vi "Laser Damage Scan Alpha.vi"(7 "Calling VI Ref":refnum<vi>) -> ()   [LabVIEW 2020]
uses:
  <vilib>/vision/Image Controls.llb/IMAQ Image.ctl
  <vilib>/Utility/miscctls.llb/LVPointTypeDef.ctl
  Display Module/Display Module Custom Controls/ROI Descriptor.ctl
  <vilib>/DAQmx/write.llb/DAQmx Write (Analog 1D Wfm NChan NSamp).vi
  <vilib>/Instr/_visa.llb/VISA Configure Serial Port (Instr).vi
  <vilib>/DAQmx/create/channels.llb/DAQmx Create Channel (AO-Voltage-Basic).vi
  <vilib>/DAQmx/configure/timing.llb/DAQmx Timing (Sample Clock).vi
  <vilib>/DAQmx/miscellaneous.llb/DAQmx Fill In Error Info.vi
  <resource>/objmgr/daqmx.rc
  <vilib>/measure/NI_MABase.lvlib
panel:
  in  "Active Image":u16(ring) items=["IDS-Camera-Primary-2", "IDS-Camera-Primary-3", "IDS-Camera-Primary-4"]
  in  "Manual Shutter":bool
  out "Current Exposure Time (s)":dbl=1.0 max=100.0 format="%.1f"
  out "Scan Error":bool
  in  "Scan Rate (Hz)":dbl=1.0 max=100.0
  in  "Exposure Time (s)":i32=1 max=100
  out "Shutter Error":bool
  in  "Ablate":bool
  out "Waveform Graph":waveform(dbl)[](graph)=[{"t0"=timestamp(0 s since 1904-01-01), "dt"=0.001, "Y"=array[100000 elements]}, {"t0"=timestamp(0 s since 1904-01-01), "dt"=0.001, "Y"=array[100000 elements]}, {"t0"=timestamp(0 s since 1904-01-01), "dt"=0.001, "Y"=array[100000 elements]}]
  in  "Quit":bool
  out "ROI Error":bool
  out "ROI Data":i32[](array[numeric])
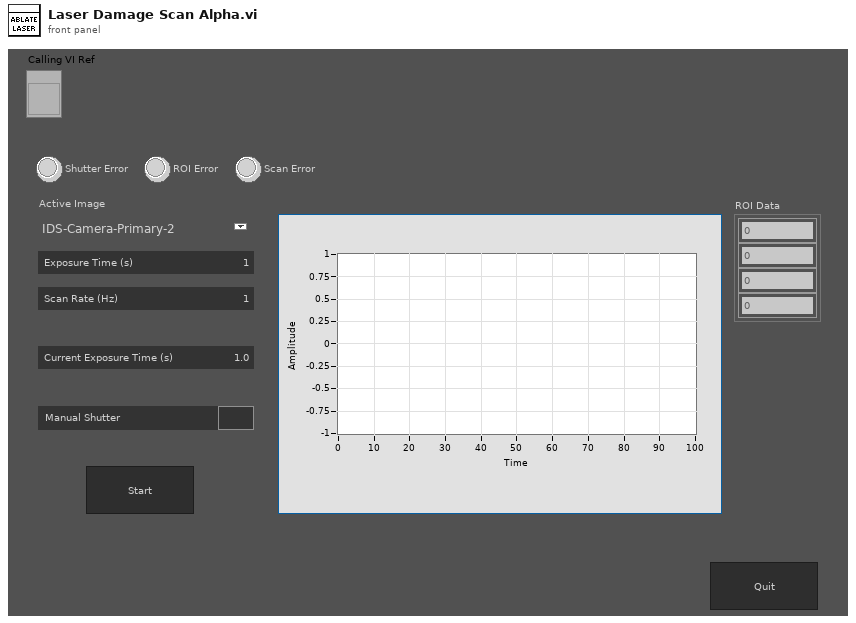
[diagram p1: front panel]
types:
  T1 = enum16{"Always On", "Always Off", "Off While Running"}
  T2 = typedef "LVPointTypeDef.ctl" = cluster{"Horizontal":i16, "Vertical":i16}
  T3 = cluster{"Vx":dbl, "Xfreq":dbl, "Xoff":dbl, "Yfreq":dbl, "Vy":dbl, "Yoff":dbl}
  T4 = typedef "IMAQ Image.ctl" = refnum<image>
  T5 = typedef "ROI Descriptor.ctl" = cluster{"Global Rectangle":i32[], "Contours":cluster{"Contour Type":u32, "ROI Type":u32, "Points":i32[]}[]}
  T6 = cluster{"Waveform Type":u16, "Amplitude":dbl, "Frequency":dbl, "Phase":dbl, "Offset":dbl}
  T7 = cluster{"Waveform Type":u16, "Amplitude":dbl, "Frequency":dbl, "Phase":dbl, "Offset":dbl}[]
  T8 = typedef "LVRectTypeDef.ctl" = cluster{"Left":i16, "Top":i16, "Right":i16, "Bottom":i16}
  T9 = typedef "LVBoundsTypeDef.ctl" = cluster{"Width":u32, "Height":u32}
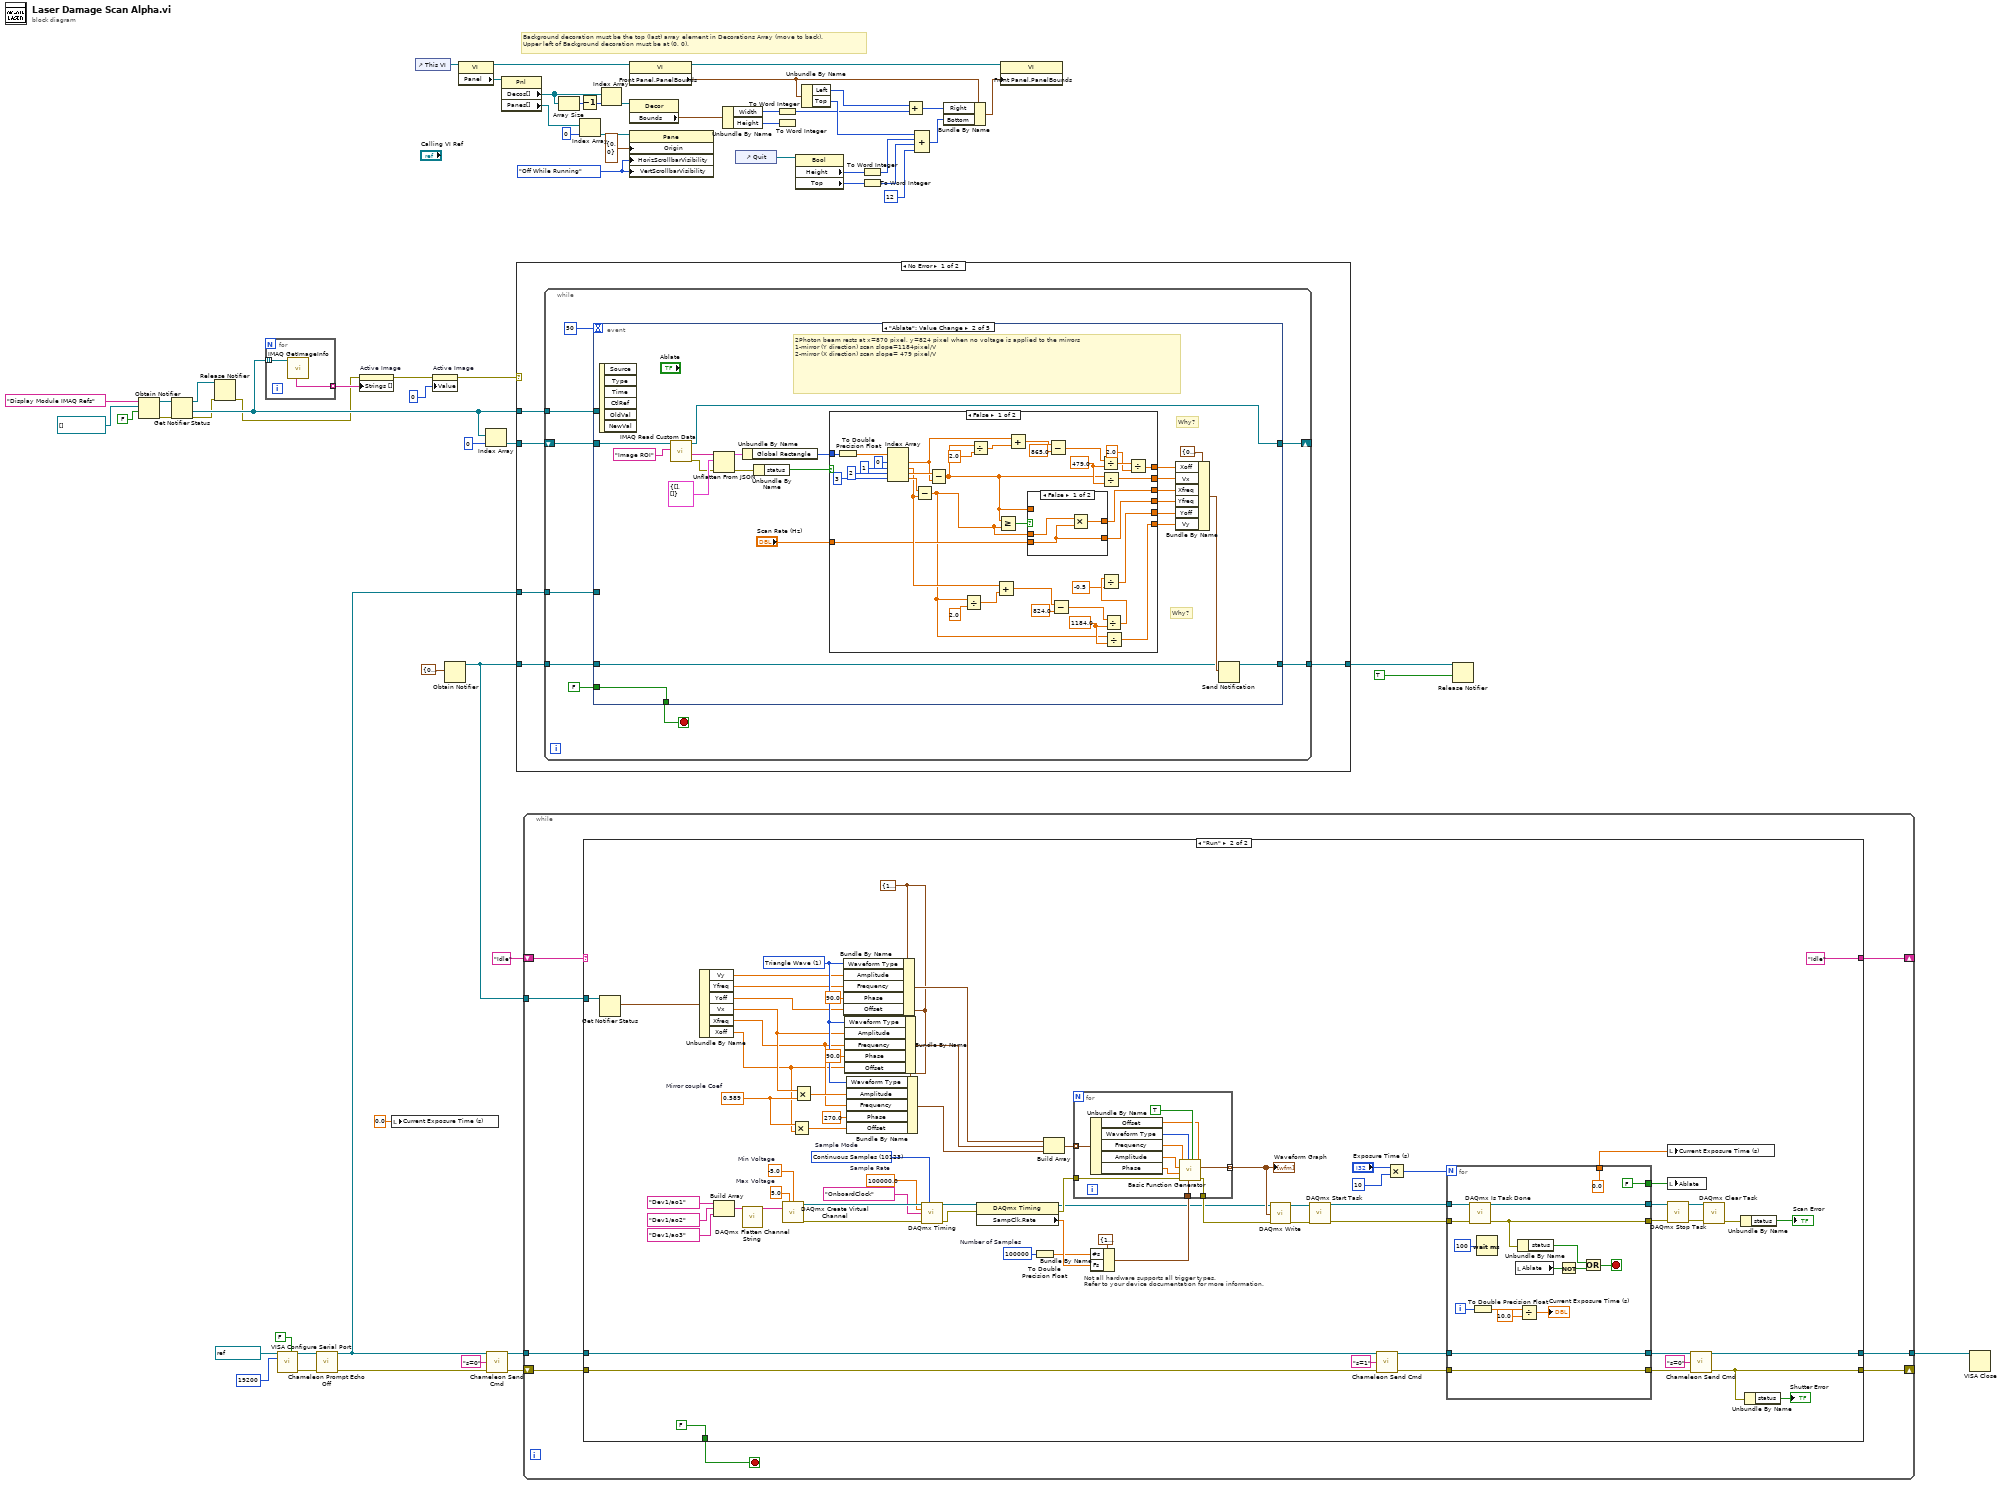
[diagram p0: block diagram]
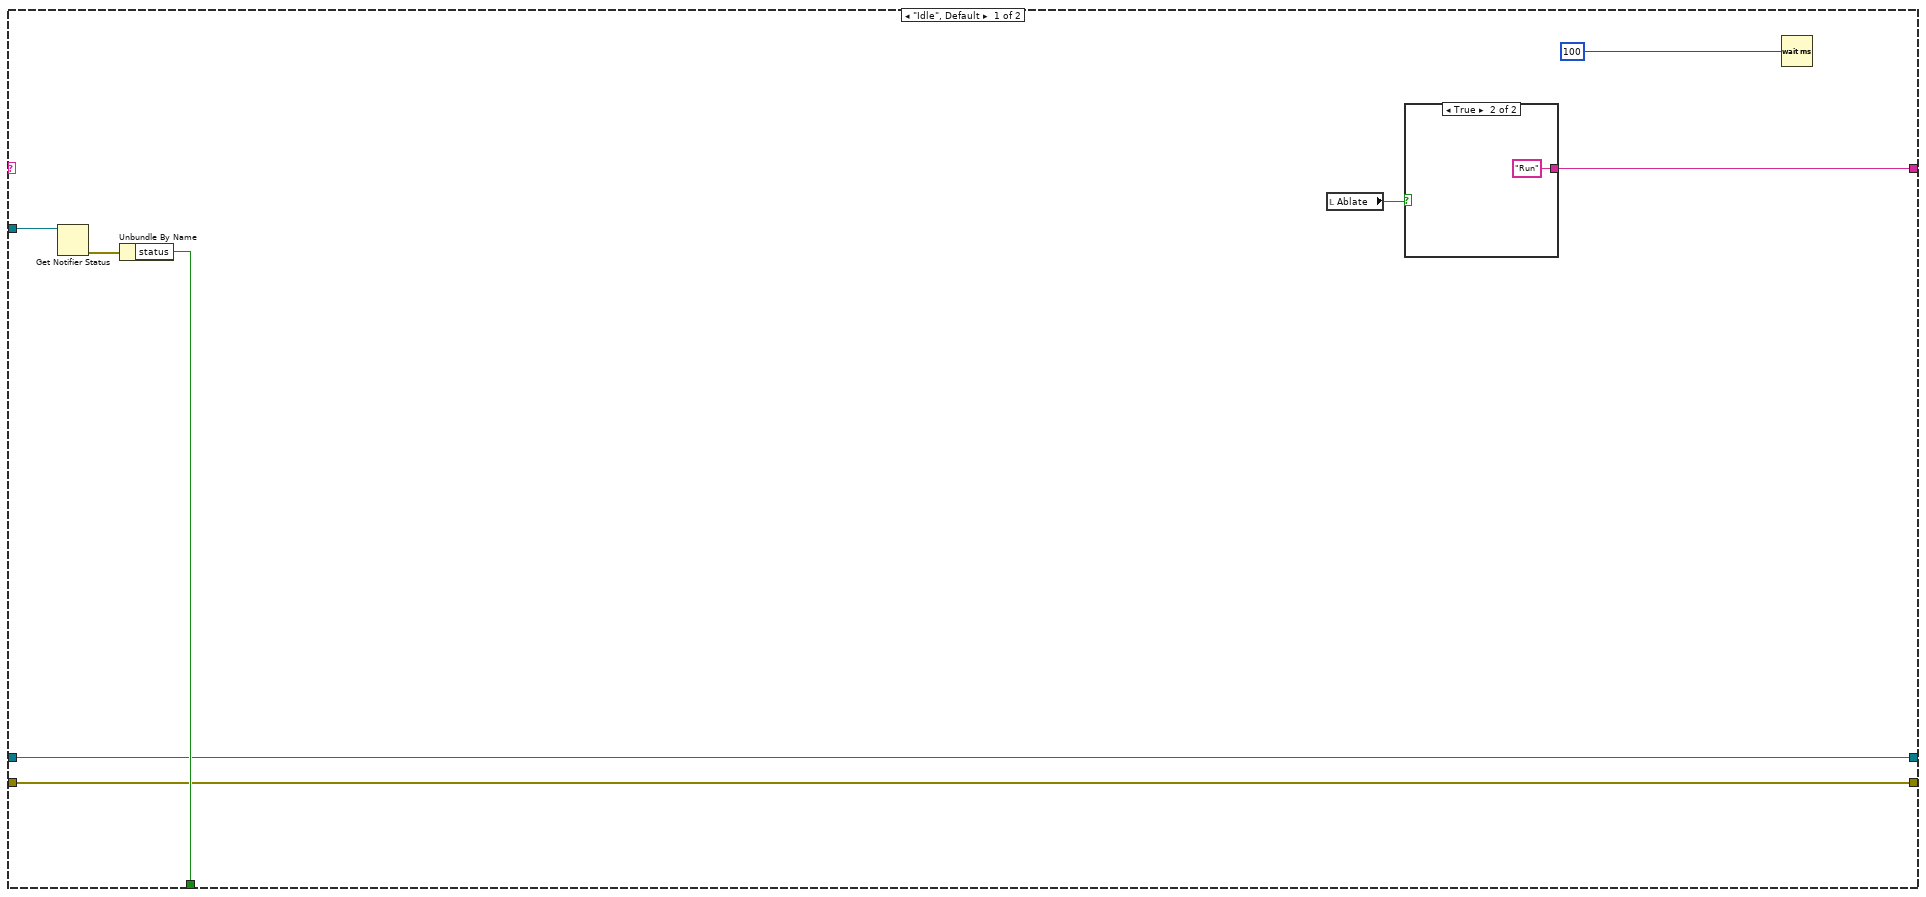
[diagram p2: hidden frame]
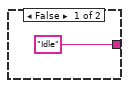
[diagram p3: hidden frame]
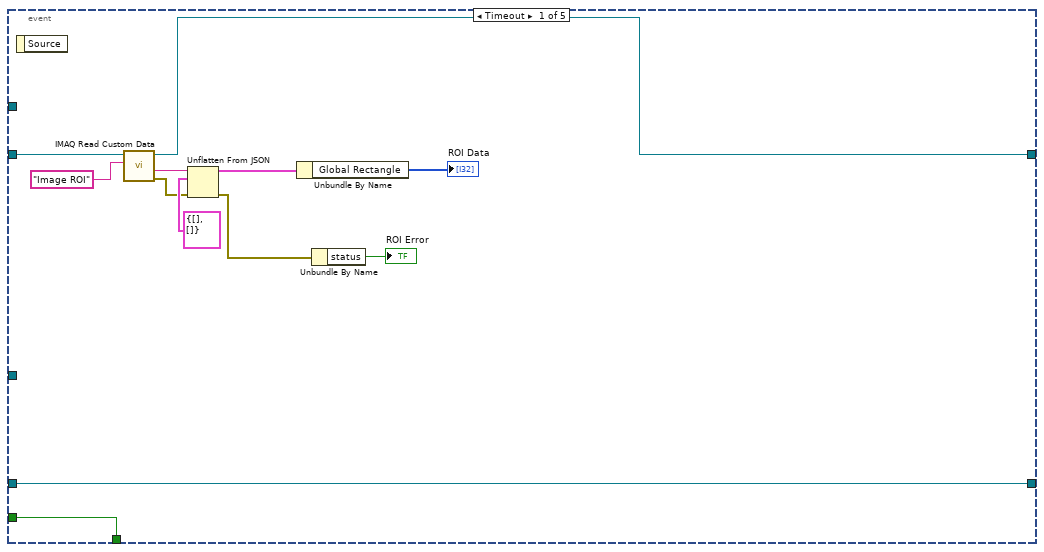
[diagram p4: hidden frame]
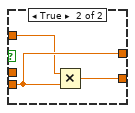
[diagram p5: hidden frame]
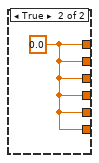
[diagram p6: hidden frame]
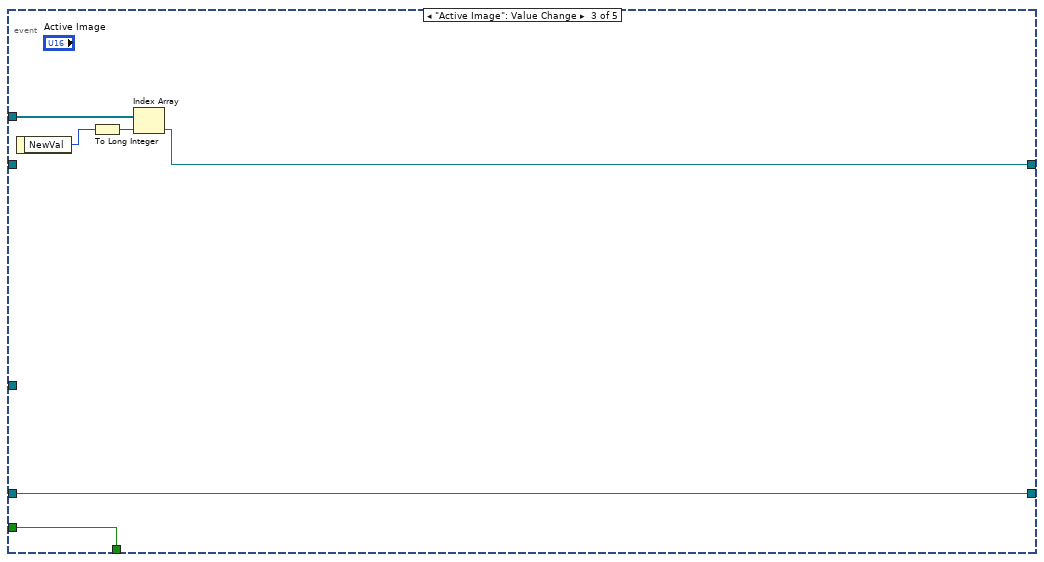
[diagram p7: hidden frame]
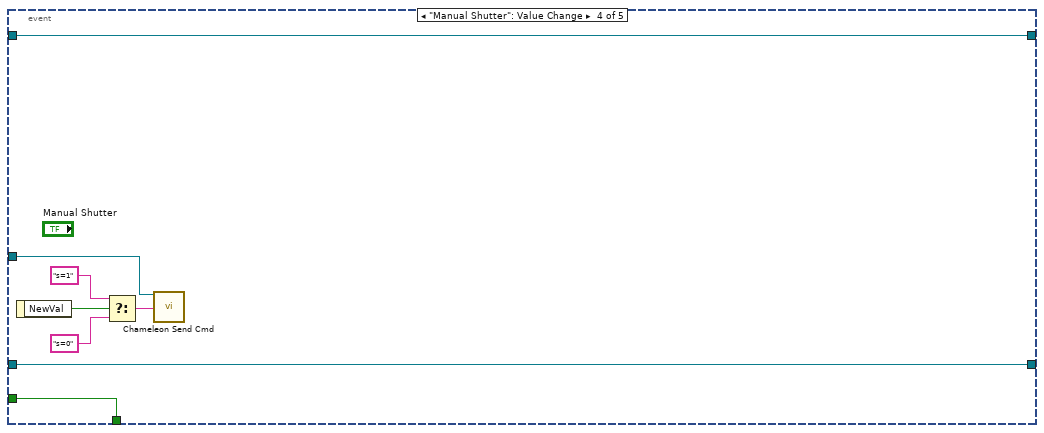
[diagram p8: hidden frame]
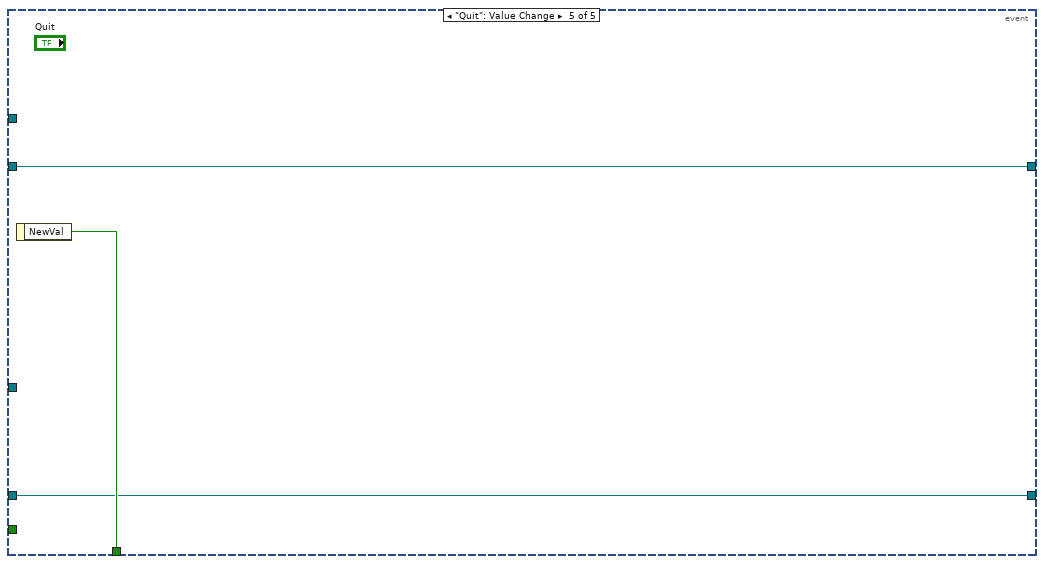
[diagram p9: hidden frame]
diagram:
  w13 = T1."Off While Running" ("Vertical Scrollbar Visibility")
  # "Background decoration must be the top (last) array element in Decorations Array (move to back).\nUpper left of Background decoration must be at (0, 0)."
  n1 = Obtain Notifier(name (unnamed)="Display Module IMAQ Refs", notification data type=T4[] [], create if not found? (T)=FALSE) -> (notifier out=w61:refnum<notifier>, error out=w60:errorcluster)  [unwired: 1 in, 1 out]
  n2 = Get Notifier Status(notifier=w61, error in (no error)=w60) -> (notifier out=w49:refnum<notifier>, current notification=w54:T4[], error out=w48:errorcluster)  [unwired: 2 out]
  n3 = Release Notifier(notifier=w49, error in (no error)=w48) -> (error out=w47:errorcluster)  [unwired: 1 in, 2 out]
  n4 = for {
    tunnel: w54 -> [w63] mode=indexing
    tunnel: [w62] -> w53 mode=indexing
    n5 = call "IMAQ GetImageInfo"("Image"=w63) -> ("Image Name"=w62:string)  [unwired: 3 in, 7 out]
  }
  n6 = call-poly "VISA Configure Serial Port"("VISA resource name"=refnum<visa-resource-name> "COM13" ("VISA Ref"), "Enable Termination\nChar (T)"=FALSE ("Enable Termination\nChar (T)"), "baud rate (9600)"=u32 19200) -> ("VISA resource name out"=w38:refnum<visa-resource-name>, "error out"=w37:errorcluster)  [unwired: 11 in]
  n7 = call "Chameleon Prompt Echo Off.vi"("VISA Ref"=w38, "Error In"=w37) -> ("VISA Ref Out"=w31:refnum<visa-resource-name>, "Error Out"=w33:errorcluster)  [unwired: 12 in]
  n8 = property on="Active Image" class="Ring (strict)"(error in=w47, "Strings []"=w53) -> (error out=w51:errorcluster)  [unwired: 1 in, 1 out]
  n9 = local write "Current Exposure Time (s)"(0.0 ("Current Exposure Time (s)")) -> ()
  n10 = control-ref of="This VI"() -> (w5:refnum<vi>)
  n11 = property on="Active Image" class="Ring (strict)"(error in=w51, "Value"=u16 0) -> (error out=w50:errorcluster)  [unwired: 1 in, 1 out]
  n12 = Obtain Notifier(notification data type=T3 {"Vx"=0.25, "Xfreq"=1.0, "Xoff"=0.1, "Yfreq"=1.0, "Vy"=0.25, "Yoff"=0.1} ("Cluster")) -> (notifier out=w43:refnum<notifier>)  [unwired: 3 in, 2 out]
  n13 = property class="VI"(reference=w5) -> (reference out=w14:refnum<vi>, "Panel"=w6:refnum<vi>)  [unwired: 1 in, 1 out]
  n14 = Index Array(array=w54, index=0) -> (element=w55:T4)
  n15 = call "Chameleon Send Cmd.vi"("VISA Ref"=w31, "Command"="s=0", "Error In"=w33) -> ("VISA Ref Out"=w34:refnum<visa-resource-name>, "Error Out"=w32:errorcluster)  [unwired: 10 in, 1 out]
  n16 = property class="Pnl"(reference=w6) -> ("Decos[]"=w4:refnum<vi>[], "Panes[]"=w10:refnum<vi>[])  [unwired: 1 in, 2 out]
  n17 = case shown="No Error" w50 {
    tunnel: w55 -> [w68 _]
    tunnel: w54 -> [w67 _]
    tunnel: w43 -> [w66 w172]
    tunnel: [w65 w172] -> w45
    tunnel: w31 -> [w64 _]
    frame No Error {
      n18 = while {
        shift-right: [w74] -> _
        shift-left: w68 -> [w75]
        tunnel: w67 -> [w76]
        tunnel: w66 -> [w71]
        tunnel: [w70] -> w65
        tunnel: w64 -> [w69]
        stop <- w72 stop-if-true
        n19 = event shown="[1] \"Ablate\": Value Change" {
          selector: _ -> [_ _ _ _ _]
          dyn-events: _ -> [_ _ _ _ _]
          timeout: 50 -> [_ _ _ _ _]
          tunnel: w76 -> [_ _ w159 _ _]
          tunnel: w75 -> [w84 w106 _ w166 w170]
          tunnel: [w83 w105 w156 w166 w170] -> w74
          tunnel: FALSE -> [w80 w104 w160 w168 _]
          tunnel: [w80 w104 w160 w168 w171] -> w72
          tunnel: w71 -> [w79 w97 w155 w167 w169]
          tunnel: [w79 w96 w155 w167 w169] -> w70
          tunnel: w69 -> [_ _ _ w161 _]
          event Timeout {
            n20 = event-data() -> ()  [unwired: 1 in, 1 out]
            n21 = call "IMAQ Read Custom Data"("Key"="Image ROI", "Image"=w84) -> ("error out"=w85:errorcluster, "Custom Data Out"=w88:string, "Image (duplicate)"=w83:T4)  [unwired: 7 in]
            n22 = Unflatten From JSON(JSON string=w88, type and defaults=T5 {"Global Rectangle"=[], "Contours"=[]} ("Image ROI Descriptor"), error in (no error)=w85) -> (value=w86:T5, error out=w82:errorcluster)  [unwired: 4 in]
            n23 = Unbundle By Name(w86) -> ("Global Rectangle"=→"ROI Data":i32[])
            n24 = Unbundle By Name(w82) -> ("status"=→"ROI Error":bool)
          }
          event "Ablate": Value Change {
            # "Why?"
            # "Why?"
            # "2Photon beam rests at x=870 pixel, y=824 pixel when no voltage is applied to the mirrors\n1-mirror (Y direction) scan slope=1184pixel/V\n2-mirror (X direction) scan slope= 479 pixel/V"
            n25 = event-data() -> ()  [unwired: 1 in, 6 out]
            n26 = call "IMAQ Read Custom Data"("Key"="Image ROI", "Image"=w106) -> ("error out"=w107:errorcluster, "Custom Data Out"=w110:string, "Image (duplicate)"=w105:T4)  [unwired: 7 in]
            n27 = Unflatten From JSON(JSON string=w110, type and defaults=T5 {"Global Rectangle"=[], "Contours"=[]} ("Image ROI Descriptor"), error in (no error)=w107) -> (value=w108:T5, error out=w92:errorcluster)  [unwired: 4 in]
            n28 = Unbundle By Name(w108) -> ("Global Rectangle"=w93:i32[])
            n29 = Unbundle By Name(w92) -> ("status"=w91:bool)
            n30 = case shown="False" w91 {
              tunnel: w93 -> [w147 _]
              tunnel: [w136 w154] -> w102
              tunnel: [w131 w154] -> w101
              tunnel: "Scan Rate (Hz)" -> [w129 _]
              tunnel: [w128 w154] -> w100
              tunnel: [w127 w154] -> w99
              tunnel: [w125 w154] -> w95
              tunnel: [w121 w154] -> w94
              frame False {
                w133 = 1184.0 ("y")
                w134 = 479.0 ("y")
                n31 = To Double Precision Float(number=w147) -> (double precision float=w120:dbl[])
                n32 = Index Array(array=w120, index #1=0 ("index"), index #2=1 ("index"), index #3=2 ("index"), index #4=3 ("index")) -> (element #1=w138:dbl, element #2=w137:dbl, element #3=w142:dbl, element #4=w140:dbl)
                n33 = Subtract(x=w140, y=w137) -> (x-y=w112:dbl)
                n34 = Subtract(x=w142, y=w138) -> (x-y=w116:dbl)
                n35 = Divide(x=w112, y=2.0) -> (x/y=w115:dbl)
                n36 = Divide(x=w116, y=2.0) -> (x/y=w119:dbl)
                n37 = Add(x=w137, y=w115) -> (x+y=w114:dbl)
                n38 = Greater Or Equal?(x=w116, y=w112) -> (x >= y?=w130:bool)
                n39 = Add(x=w138, y=w119) -> (x+y=w118:dbl)
                n40 = case shown="False" w130 {
                  tunnel: w129 -> [w150 w152]
                  tunnel: [w150 w153] -> w128
                  tunnel: w112 -> [w148 _]
                  tunnel: [w149 w152] -> w127
                  tunnel: w116 -> [_ w151]
                  frame False {
                    n41 = Multiply(x=w148, y=w150) -> (x*y=w149:dbl)
                  }
                  frame True {
                    n42 = Multiply(x=w151, y=w152) -> (x*y=w153:dbl)
                  }
                }
                n43 = Subtract(x=w118, y=865.0) -> (x-y=w117:dbl)
                n44 = Subtract(x=w114, y=824.0) -> (x-y=w113:dbl)
                n45 = Divide(x=w117, y=w134) -> (x/y=w126:dbl)
                n46 = Divide(x=w116, y=w134) -> (x/y=w136:dbl)
                n47 = Divide(x=w113, y=w133) -> (x/y=w123:dbl)
                n48 = Divide(x=w123, y=-0.5) -> (x/y=w121:dbl)
                n49 = Divide(x=w112, y=w133) -> (x/y=w131:dbl)
                n50 = Divide(x=w126, y=2.0) -> (x/y=w125:dbl)
              }
              frame True {
                w154 = 0.0
              }
            }
            n51 = Bundle By Name(cluster=T3 {"Vx"=0.25, "Xfreq"=1.0, "Xoff"=0.1, "Yfreq"=1.0, "Vy"=0.25, "Yoff"=0.1} ("Cluster"), "Xoff"=w95, "Vx"=w102, "Xfreq"=w99, "Yfreq"=w100, "Yoff"=w94, "Vy"=w101) -> (w98:T3)
            n52 = Send Notification(notification=w98, notifier=w97) -> (notifier out=w96:refnum<notifier>)  [unwired: 1 in, 1 out]
          }
          event "Active Image": Value Change {
            n53 = event-data() -> ("NewVal"=w158:u16)  [unwired: 1 in]
            n54 = To Long Integer(number=w158) -> (32bit integer=w157:i32)
            n55 = Index Array(array=w159, index=w157) -> (element=w156:T4)
          }
          event "Manual Shutter": Value Change {
            n56 = event-data() -> ("NewVal"=w165:bool)  [unwired: 1 in]
            n57 = Select(t="s=1" ("Command"), s=w165, f="s=0" ("Command")) -> (s? t:f=w162:string)
            n58 = call "Chameleon Send Cmd.vi"("VISA Ref"=w161, "Command"=w162) -> ()  [unwired: 11 in, 3 out]
          }
          event "Quit": Value Change {
            n59 = event-data() -> ("NewVal"=w171:bool)  [unwired: 1 in]
          }
        }
      }
    }
    frame Error {
    }
  }
  n60 = while {
    tunnel: w43 -> [w179]
    shift-right: [w178] -> _
    shift-left: "Idle" -> [w177]
    shift-right: [w173] -> _
    shift-left: w32 -> [w176]
    tunnel: w34 -> [w175]
    tunnel: [w174] -> w36
    stop <- w180 stop-if-true
    n61 = case shown="\"Run\"" w177 {
      tunnel: [w186 FALSE] -> w180
      tunnel: w179 -> [w188 w216]
      tunnel: [w184 "Idle"] -> w178
      tunnel: w176 -> [w181 w207]
      tunnel: w175 -> [w182 w208]
      tunnel: [w182 w206] -> w174
      tunnel: [w181 w205] -> w173
      frame "Idle", Default {
        n62 = Get Notifier Status(notifier=w188) -> (error out=w187:errorcluster)  [unwired: 1 in, 4 out]
        n63 = Unbundle By Name(w187) -> ("status"=w186:bool)
        n64 = local read "Ablate"() -> (w185:bool)
        n65 = case shown="True" w185 {
          tunnel: ["Idle" "Run"] -> w184
          frame False {
          }
          frame True {
          }
        }
        n66 = Wait (ms)(milliseconds to wait=u32 100) -> ()  [unwired: 1 out]
      }
      frame "Run" {
        w242 = 100000  # Number of Samples
        w220 = 0.589  # Mirror couple Coef
        w251 = 5.0  # Max Voltage
        w252 = -5.0  # Min Voltage
        w225 = u16 1 items=["Sine Wave", "Triangle Wave", "Square Wave", "Sawtooth Wave"] ("Waveform Type")
        w226 = T6 {"Waveform Type"=1, "Amplitude"=0.25, "Frequency"=1.0, "Phase"=180.0, "Offset"=0.1} ("Cluster")
        w253 = 100000.0  # Sample Rate
        w259 = 10123 items=["Finite Samples"=10178, "Continuous Samples"=10123, "Hardware Timed Single Point"=12522]  # Sample Mode
        # "Not all hardware supports all trigger types.\nRefer to your device documentation for more information."
        n67 = Get Notifier Status(notifier=w216) -> (current notification=w215:T3)  [unwired: 1 in, 4 out]
        n68 = Unbundle By Name(w215) -> ("Vy"=w214:dbl, "Yfreq"=w213:dbl, "Yoff"=w212:dbl, "Vx"=w211:dbl, "Xfreq"=w210:dbl, "Xoff"=w209:dbl)
        n69 = Build Array(tag "Dev1/ao1" ("Physical Channel(s)"), tag "Dev1/ao2" ("Physical Channel(s)"), tag "Dev1/ao3" ("Physical Channel(s)")) -> (w234:tag[])
        n70 = call <vilib>:"DAQmx Flatten Channel String.vi"("names in"=w234) -> ("names out"=w231:string)  [unwired: 13 in, 1 out]
        n71 = call-poly <vilib>:"DAQmx Create Virtual Channel.vi"("maximum value"=w251, "minimum value"=w252, "physical channels"=w231) -> ("task out"=w257:refnum<k21>, "error out"=w258:errorcluster)  [unwired: 11 in]
        n72 = Multiply(x=w220, y=w209) -> (x*y=w219:dbl)
        n73 = Multiply(x=w211, y=w220) -> (x*y=w221:dbl)
        n74 = Bundle By Name(cluster=w226, "Waveform Type"=w225, "Amplitude"=w214, "Frequency"=w213, "Phase"=90.0, "Offset"=w212) -> (w229:T6)
        n75 = Bundle By Name(cluster=w226, "Waveform Type"=w225, "Amplitude"=w211, "Frequency"=w210, "Phase"=90.0, "Offset"=w209) -> (w228:T6)
        n76 = Bundle By Name(cluster=w226, "Waveform Type"=w225, "Amplitude"=w221, "Frequency"=w210, "Phase"=270.0, "Offset"=w219) -> (w227:T6)
        n77 = call-poly <vilib>:"DAQmx Timing.vi"("task/channels in"=w257, "sample mode"=w259, "rate"=w253, "source"=tag "OnboardClock" ("Sample Clock Source"), "error in"=w258) -> ("task out"=w261:refnum<k21>, "error out"=w260:errorcluster)  [unwired: 9 in]
        n78 = property class="DAQmx Timing"(reference=w261, error in=w260) -> (reference out=w236:refnum<k21>, error out=w237:errorcluster, "SampClk.Rate"=w249:dbl)
        n79 = To Double Precision Float(number=w242) -> (double precision float=w243:dbl)
        n80 = Build Array(w229, w228, w227) -> (w230:T7)
        n81 = Bundle By Name(cluster=cluster{"Fs":dbl, "#s":dbl} {"Fs"=1000.0, "#s"=1000.0} ("sampling info"), "#s"=w243, "Fs"=w249) -> (w248:cluster{"Fs":dbl, "#s":dbl})
        n82 = for {
          tunnel: w237 -> [w289]
          tunnel: w248 -> [w288]
          tunnel: [w287] -> w245
          tunnel: w230 -> [w286] mode=indexing
          tunnel: [w282] -> w244 mode=indexing
          n83 = Unbundle By Name(w286) -> ("Offset"=w279:dbl, "Waveform Type"=w285:u16, "Frequency"=w284:dbl, "Amplitude"=w283:dbl, "Phase"=w281:dbl)
          n84 = call <vilib>:"Basic Function Generator.vi"("offset"=w279, "reset signal"=TRUE, "sampling info"=w288, "signal type"=w285, "error in (no error)"=w289, "phase"=w281, "amplitude"=w283, "frequency"=w284) -> ("error out"=w287:errorcluster, "signal out"=w282:waveform(dbl))  [unwired: 1 in, 1 out]
        }
        "Waveform Graph" <- w244
        n85 = call-poly <vilib>:"DAQmx Write.vi"("task/channels in"=w236, "data"=w244, "error in"=w245) -> ("task out"=w247:refnum<k21>, "error out"=w246:errorcluster)  [unwired: 10 in, 1 out]
        n86 = call <vilib>:"DAQmx Start Task.vi"("task/channels in"=w247, "error in"=w246) -> ("task out"=w256:refnum<k21>, "error out"=w255:errorcluster)  [unwired: 12 in]
        n87 = call "Chameleon Send Cmd.vi"("VISA Ref"=w208, "Command"="s=1", "Error In"=w207) -> ("VISA Ref Out"=w200:refnum<visa-resource-name>, "Error Out"=w199:errorcluster)  [unwired: 10 in, 1 out]
        n88 = Multiply(x="Exposure Time (s)", y=10) -> (x*y=w195:i32)
        n89 = for {
          N: w195 -> [_]
          tunnel: w256 -> [w278]
          tunnel: w255 -> [w277]
          tunnel: [w275] -> w238
          tunnel: [w276] -> w239
          tunnel: [w272] -> w201
          tunnel: w200 -> [w272]
          tunnel: w199 -> [w271]
          tunnel: [w271] -> w198
          tunnel: [FALSE] -> w194
          tunnel: [0.0] -> w191
          i -> [w266]
          stop <- w268 stop-if-true
          n90 = call <vilib>:"DAQmx Is Task Done.vi"("task/channels in"=w278, "error in"=w277) -> ("task out"=w276:refnum<k21>, "error out"=w275:errorcluster)  [unwired: 11 in, 1 out]
          n91 = To Double Precision Float(number=w266) -> (double precision float=w265:dbl)
          n92 = Wait (ms)(milliseconds to wait=u32 100) -> ()  [unwired: 1 out]
          n93 = local read "Ablate"() -> (w274:bool)
          n94 = Unbundle By Name(w275) -> ("status"=w270:bool)
          n95 = Divide(x=w265, y=10.0) -> (x/y=→"Current Exposure Time (s)":dbl)
          n96 = Not(x=w274) -> (.not. x?=w269:bool)
          n97 = Or(x=w270, y=w269) -> (x .or. y?=w268:bool)
        }
        n98 = local write "Current Exposure Time (s)"(w191) -> ()
        n99 = local write "Ablate"(w194) -> ()
        n100 = call <vilib>:"DAQmx Stop Task.vi"("task/channels in"=w239, "error in"=w238) -> ("task out"=w241:refnum<k21>, "error out"=w240:errorcluster)  [unwired: 12 in]
        n101 = call "Chameleon Send Cmd.vi"("VISA Ref"=w201, "Command"="s=0", "Error In"=w198) -> ("VISA Ref Out"=w206:refnum<visa-resource-name>, "Error Out"=w205:errorcluster)  [unwired: 10 in, 1 out]
        n102 = call <vilib>:"DAQmx Clear Task.vi"("task in"=w241, "error in"=w240) -> ("error out"=w193:errorcluster)  [unwired: 13 in]
        n103 = Unbundle By Name(w193) -> ("status"=→"Scan Error":bool)
        n104 = Unbundle By Name(w205) -> ("status"=→"Shutter Error":bool)
      }
    }
  }
  n105 = Array Size(array=w4) -> (size(s)=w2:i32)
  n106 = Decrement(x=w2) -> (x-1=w3:i32)
  n107 = Index Array(array=w10, index=0) -> (element=w9:refnum<vi>)
  n108 = Index Array(array=w4, index=w3) -> (element=w12:refnum<vi>)
  n109 = property class="VI"(reference=w14) -> (reference out=w16:refnum<vi>, "Front Panel.PanelBounds"=w17:T8)  [unwired: 1 in, 1 out]
  n110 = property class="Decor"(reference=w12) -> ("Bounds"=w15:T9)  [unwired: 1 in, 2 out]
  n111 = property class="Pane"(reference=w9, "Origin"=T2 {"Horizontal"=0, "Vertical"=0}, "HorizScrollbarVisibility"=w13, "VertScrollbarVisibility"=w13) -> ()  [unwired: 1 in, 2 out]
  n112 = Unbundle By Name(w15) -> ("Width"=w20:u32, "Height"=w23:u32)
  n113 = control-ref of="Quit"() -> (w7:refnum<vi>)
  n114 = To Word Integer(number=w20) -> (16bit integer=w22:i16)
  n115 = To Word Integer(number=w23) -> ()  [unwired: 1 out]
  n116 = property class="Bool"(reference=w7) -> ("Height"=w25:u32, "Top"=w26:i32)  [unwired: 1 in, 2 out]
  n117 = Unbundle By Name(w17) -> ("Left"=w19:i16, "Top"=w30:i16)
  n118 = To Word Integer(number=w25) -> (16bit integer=w28:i16)
  n119 = To Word Integer(number=w26) -> (16bit integer=w29:i16)
  n120 = Add(x=w19, y=w22) -> (x+y=w21:i16)
  n121 = Compound Arithmetic op=ADD(w30, w28, w29, i16 12 ("y")) -> (w24:i16)
  n122 = Bundle By Name(cluster=w17, "Right"=w21, "Bottom"=w24) -> (w18:T8)
  n123 = property class="VI"(reference=w16, "Front Panel.PanelBounds"=w18) -> ()  [unwired: 1 in, 2 out]
  n124 = Release Notifier(notifier=w45, force destroy? (F)=TRUE) -> ()  [unwired: 1 in, 3 out]
  n125 = VISA Close(VISA resource name=w36) -> ()  [unwired: 1 in, 1 out]
